vi "ReadWrite.Data.Write.vi"(8 "error in":errorcluster, 9 "Offset":i32, 10 "Values":dbl[](array[numeric]), 11 "Ref":T1) -> (0 "error out":errorcluster)   [LabVIEW 2024, in "VS Plugin Data Access Engine.lvlib" / "Plugin Data Access Engine.lvclass"]
uses:
  Plugin Data Access Engine.lvclass
  Types/ReadWrite.DVR.ctl
  Access Type Classes/ReadWrite/ReadWrite.lvclass
  Plugin Data Access Engine.lvclass/Plugin Data Access Engine.ctl
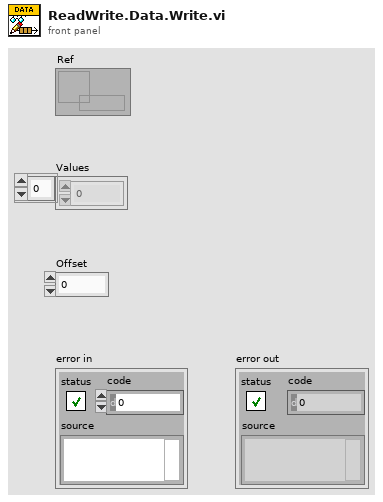
[diagram p1: front panel]
types:
  T1 = typedef "VS Plugin Data Access Engine.lvlib/Plugin Data Access Engine.lvclass/ReadWrite.DVR.ctl" = refnum<data-value>
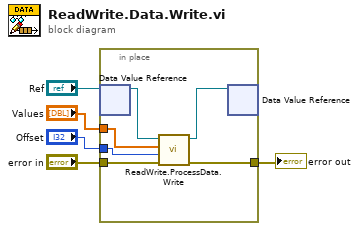
[diagram p0: block diagram]
diagram:
  n1 = in-place {
    in-place-border: "error in" -> [w11]
    in-place-border: [w10] -> w4
    in-place-border: "Values" -> [w7]
    in-place-border: "Offset" -> [w6]
    n2 = in-place-dvr #1("Ref") -> (w9:refnum<class "ReadWrite.lvclass">)  [unwired: 1 out]
    n3 = call "ReadWrite.ProcessData.Write.vi"("error in"=w11, "Offset"=w6, "Values"=w7, "ReadWrite in"=w9) -> ("error out"=w10:errorcluster, "ReadWrite out"=w8:refnum<class "ReadWrite.lvclass">)  [unwired: 6 in]
    n4 = in-place-dvr #1(w8) -> ()  [unwired: 2 out]
  }
  "error out" <- w4
